vi "Quote and Escape JSON string.vi"(11 "Plain Text":string) -> (3 "<JSON>":string caption="JSON string (quoted and escaped)")   [LabVIEW 2020, in "Library Commun.lvlib" / "JSON support.lvlib"]
uses:
  support/JSON support.lvlib
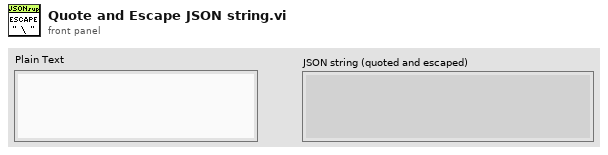
[diagram p1: front panel]
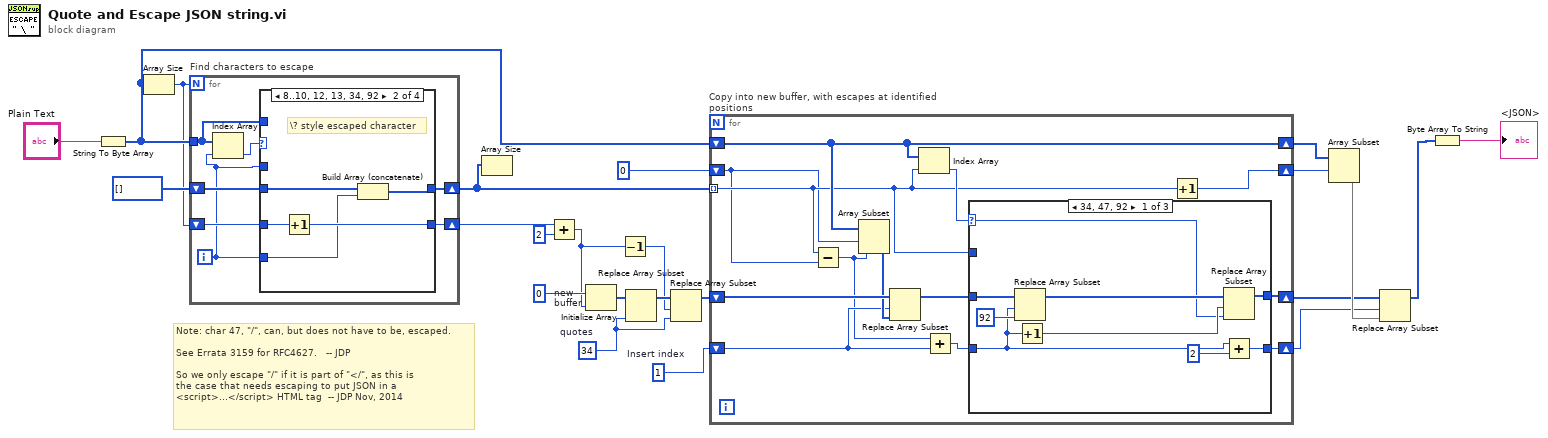
[diagram p0: block diagram]
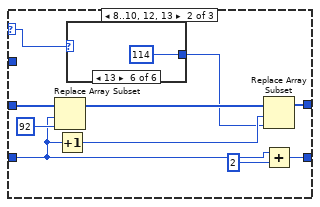
[diagram p2: hidden frame]
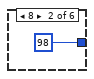
[diagram p4: hidden frame]
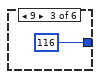
[diagram p5: hidden frame]
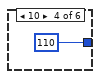
[diagram p6: hidden frame]
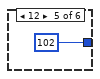
[diagram p7: hidden frame]
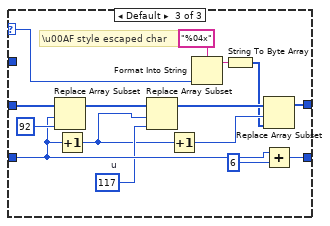
[diagram p8: hidden frame]
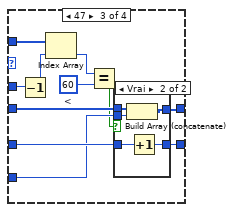
[diagram p10: hidden frame]
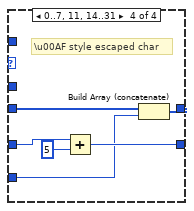
[diagram p12: hidden frame]
diagram:
  w3 = u8 34  # quotes
  w13 = 1  # Insert index
  # "Note: char 47, \"/\", can, but does not have to be, escaped.\n\nSee Errata 3159 for RFC4627.   -- JDP\n\nSo we only escape \"/\" if it is part of \"</\", as this is\nthe case that needs escaping to put JSON in a\n<script>...</script> HTML tag  -- JDP Nov, 2014"
  n1 = String To Byte Array(string="Plain Text") -> (unsigned byte array=w17:u8[])
  n2 = Array Size(array=w17) -> (size(s)=w16:i32)
  n3 = for "Find characters to escape" {
    N: w16 -> [_]
    tunnel: w17 -> [w25]
    shift-right: [w29] -> w20
    shift-left: w16 -> [w30]
    shift-right: [w28] -> w18
    shift-left: i32[] [] -> [w27]
    i -> [w24]
    n4 = Index Array(array=w25, index=w24) -> (element=w26:u8)
    n5 = case shown="8..10, 12, 13, 34, 92" w26 {
      tunnel: w30 -> [w32 w37 w48 w58]
      tunnel: [w32 w36 w47 w61] -> w29
      tunnel: [w31 w35 w46 w60] -> w28
      tunnel: w27 -> [w31 w34 w45 w59]
      tunnel: w24 -> [_ w33 w44 w56]
      tunnel: w25 -> [_ _ w41 _]
      tunnel: w24 -> [_ _ w43 _]
      frame Default {
        # "Not escaped"
      }
      frame 8..10, 12, 13, 34, 92 {
        # "\\? style escaped character"
        n6 = Increment(x=w37) -> (x+1=w36:i32)
        n7 = Build Array (concatenate)(w34, w33) -> (w35:i32[])
      }
      frame 47 {
        w39 = u8 60  # <
        n8 = Decrement(x=w43) -> (x-1=w42:i32)
        n9 = Index Array(array=w41, index=w42) -> (element=w40:u8)
        n10 = Equal?(x=w40, y=w39) -> (x = y?=w38:bool)
        n11 = case shown="Vrai" w38 {
          tunnel: w48 -> [w49 w55]
          tunnel: [w49 w54] -> w47
          tunnel: [w50 w53] -> w46
          tunnel: w45 -> [w50 w52]
          tunnel: w44 -> [_ w51]
          frame False {
          }
          frame True {
            n12 = Build Array (concatenate)(w52, w51) -> (w53:i32[])
            n13 = Increment(x=w55) -> (x+1=w54:i32)
          }
        }
      }
      frame 0..7, 11, 14..31 {
        # "\\u00AF style escaped char"
        n14 = Add(x=w58, y=5) -> (x+y=w61:i32)
        n15 = Build Array (concatenate)(w59, w56) -> (w60:i32[])
      }
    }
  }
  n16 = Array Size(array=w18) -> ()  [unwired: 1 out]
  n17 = Add(x=w20, y=2) -> (x+y=w5:i32)
  n18 = Initialize Array "new\nbuffer"(u8 0, w5) -> (w14:u8[])
  n19 = Decrement(x=w5) -> (x-1=w4:i32)
  n20 = Replace Array Subset(array=w14, new element=w3) -> (w7:u8[])  [unwired: 1 in]
  n21 = Replace Array Subset(array=w7, new element=w3, index=w4) -> (w6:u8[])
  n22 = for "Copy into new buffer, with escapes at identified positions" {
    tunnel: w18 -> [w64] mode=indexing
    shift-right: [w69] -> w10
    shift-left: w17 -> [w69]
    shift-right: [w68] -> w9
    shift-left: w13 -> [w67]
    shift-right: [w70] -> w11
    shift-left: w6 -> [w73]
    shift-right: [w62] -> w1
    shift-left: 0 -> [w63]
    n23 = Subtract(x=w64, y=w63) -> (x-y=w65:i32)
    n24 = Array Subset(array=w69, index=w63, length=w65) -> (w72:u8[])
    n25 = Replace Array Subset(array=w73, new element=w72, index=w67) -> (w71:u8[])
    n26 = Index Array(array=w69, index=w64) -> (element=w74:u8)
    n27 = Add(x=w65, y=w67) -> (x+y=w66:i32)
    n28 = case shown="34, 47, 92" w74 {
      selector: w74 -> [w79 w85 w105]
      tunnel: w71 -> [w83 w93 w113]
      tunnel: w64 -> [_ _ _]
      tunnel: [w78 w89 w111] -> w70
      tunnel: w66 -> [w75 w86 w108]
      tunnel: [w76 w87 w109] -> w68
      frame 34, 47, 92 {
        n29 = Replace Array Subset(array=w83, new element=u8 92 ("new element/subarray"), index=w75) -> (w81:u8[])
        n30 = Increment(x=w75) -> (x+1=w80:i32)
        n31 = Replace Array Subset(array=w81, new element=w79, index=w80) -> (w78:u8[])
        n32 = Add(x=w75, y=2) -> (x+y=w76:i32)
      }
      frame 8..10, 12, 13 {
        n33 = Replace Array Subset(array=w93, new element=u8 92 ("new element/subarray"), index=w86) -> (w91:u8[])
        n34 = Increment(x=w86) -> (x+1=w90:i32)
        n35 = case shown="13" w85 {
          tunnel: [_ u8 98 u8 116 u8 110 u8 102 u8 114] -> w84
          frame 0, Default {
          }
          frame 8 {
          }
          frame 9 {
          }
          frame 10 {
          }
          frame 12 {
          }
          frame 13 {
          }
        }
        n36 = Replace Array Subset(array=w91, new element=w84, index=w90) -> (w89:u8[])
        n37 = Add(x=w86, y=2) -> (x+y=w87:i32)
      }
      frame Default {
        w104 = u8 117  # u
        # "\\u00AF style escaped char"
        n38 = Replace Array Subset(array=w113, new element=u8 92 ("new element/subarray"), index=w108) -> (w103:u8[])
        n39 = Increment(x=w108) -> (x+1=w101:i32)
        n40 = Replace Array Subset(array=w103, new element=w104, index=w101) -> (w102:u8[])
        n41 = Increment(x=w101) -> (x+1=w100:i32)
        n42 = Format Into String(format string="%04x", w105) -> (resulting string=w106:string)  [unwired: 2 in, 1 out]
        n43 = String To Byte Array(string=w106) -> (unsigned byte array=w99:u8[])
        n44 = Replace Array Subset(array=w102, new element=w99, index=w100) -> (w111:u8[])
        n45 = Add(x=w108, y=6) -> (x+y=w109:i32)
      }
    }
    n46 = Increment(x=w64) -> (x+1=w62:i32)
  }
  n47 = Array Subset(array=w10, index=w1) -> (w12:u8[])  [unwired: 1 in]
  n48 = Replace Array Subset(array=w11, new element=w12, index=w9) -> (w19:u8[])
  n49 = Byte Array To String(unsigned byte array=w19) -> (string=→"<JSON>":string)
